vi "ATR.vi"() -> ()   [LabVIEW 2017]
panel:
  out "ATR 2":string[][](table)=[["Test Communication", "-", "-", "-", "-", ""], ["Set S/N", "-", "-", "-", "-", ""], ["Set Board Number", "-", "-", "-", "-", ""], [" ", "", "", "", "", ""], ["Test Communication", "-", "-", "-", "-", ""], ["Get S/N", "-", "-", "-", "", ""], ["Get Board Number", "-", "-", "-", "", ""], ["Get FW", "-", "-", "-", "", ""], ["Enable Motor", "", "", "", "", ""], ["Small position command", "", "", "", "", ""], ["Measure delta", "", "", "", "", ""], ["Velocity command", "", "", "", "", ""]] caption="ATR"
  out "ATR":string[][](table)=[["Test Communication", "-", "-", "-", "-", ""], ["Set S/N", "-", "-", "-", "-", ""], ["Set Board Number", "-", "-", "-", "-", ""], [" ", "", "", "", "", ""], ["Test Communication", "-", "-", "-", "-", ""], ["Get S/N", "-", "-", "-", "", ""], ["Get Board Number", "-", "-", "-", "", ""], ["Get FW", "-", "-", "-", "", ""], ["Enable Motor", "", "", "", "", ""], ["Small position command", "", "", "", "", ""], ["Measure delta", "", "", "", "", ""], ["Velocity command", "", "", "", "", ""]]
  out "Array 2":string[](array[string])
  out "Array":string[](array[string])
  out "deleted portion 2":string[](array[string])
  out "deleted portion":string[](array[string])
  out "ArrAHU":string[][](array[string])
  out "ArrEbay":string[][](array[string])
  out "Mort Temp":string[][](array[string])
  out "Aux":string[][](array[string])
  out "Burnin":string[][](array[string])
  out "Temp Algo":string[][](array[string])
  out "Speed":string[][](array[string])
  out "Tempreature calibration":string[][](array[string])
  out "StopTime":string[][](array[string])
  out "Enable":string[][](array[string])
  out "Communication":string[][](array[string])
  out "Visual Inspection":string[][](array[string])
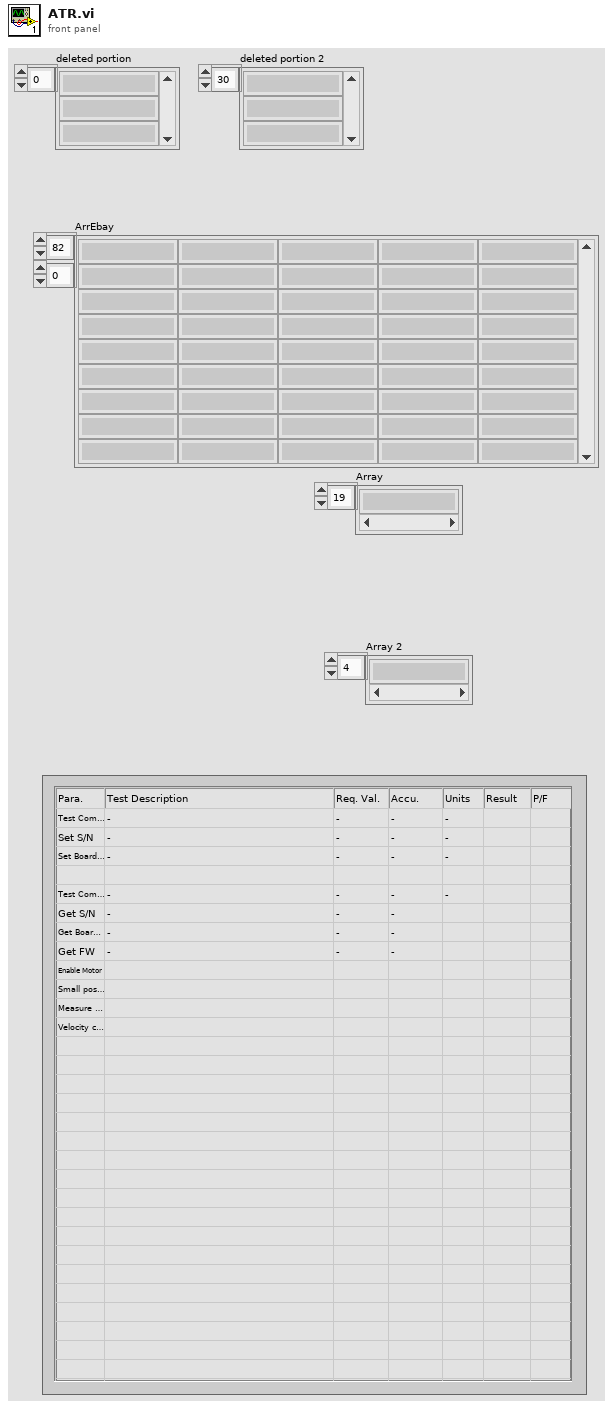
[diagram p1: front panel]
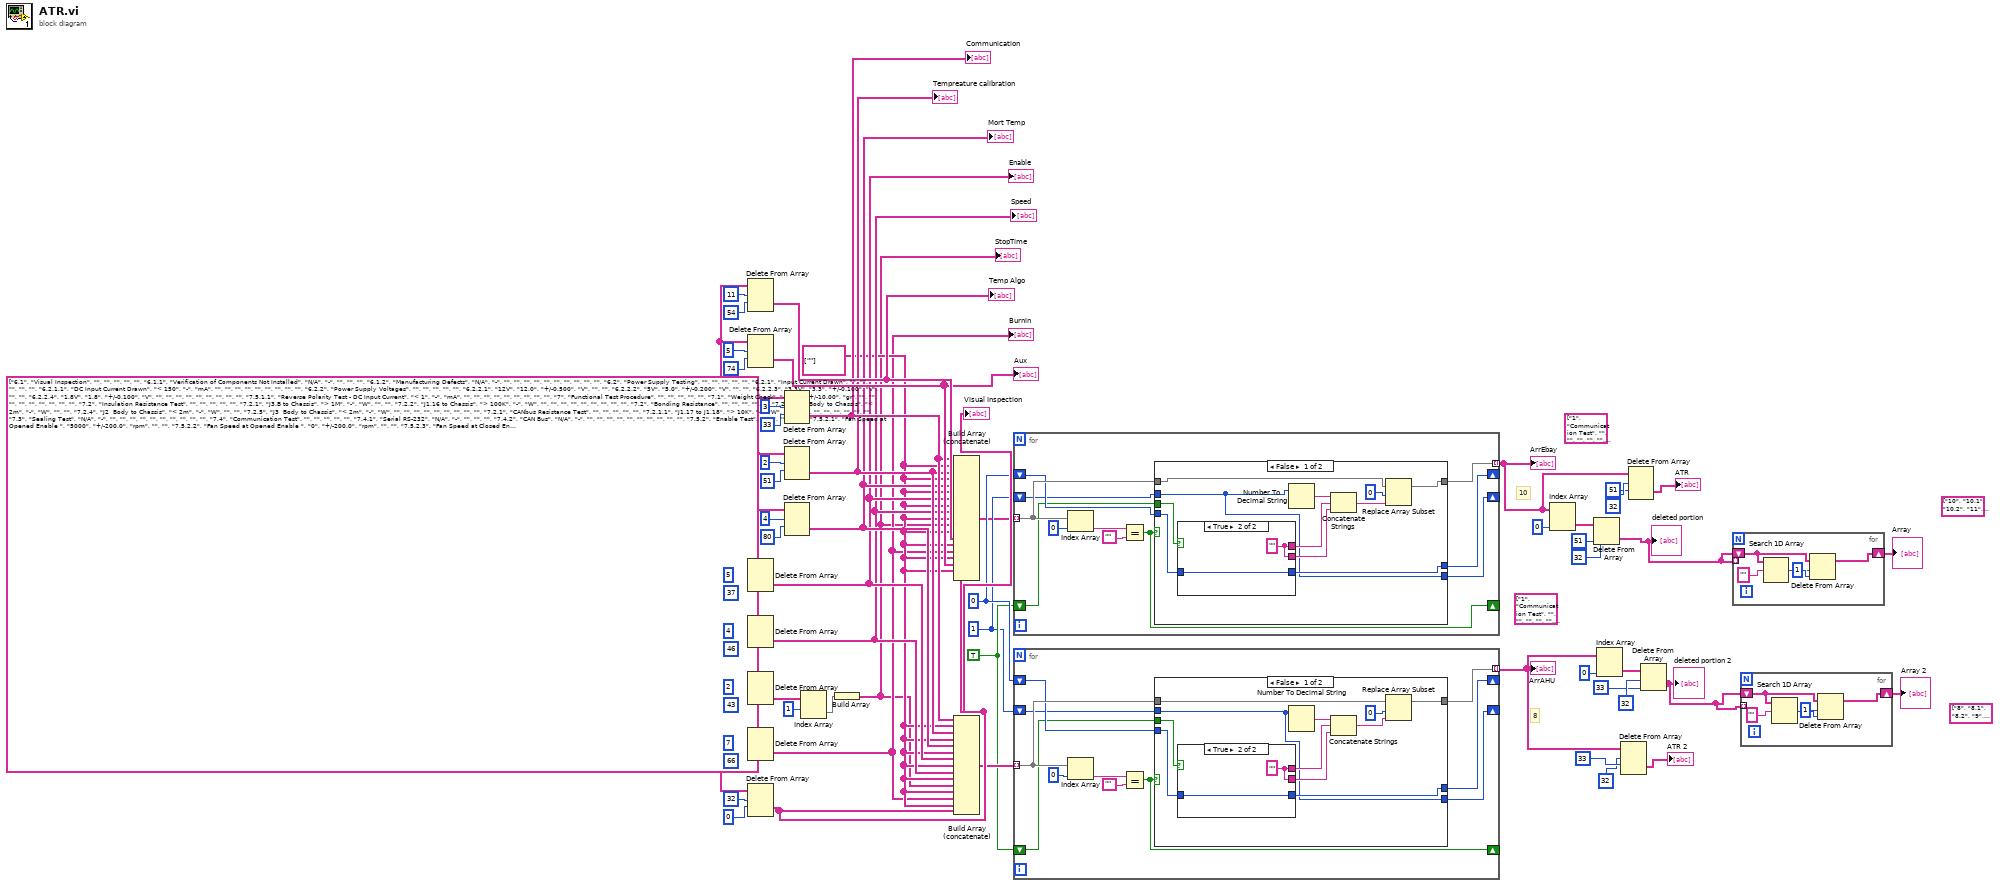
[diagram p0: block diagram]
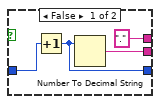
[diagram p2: hidden frame]
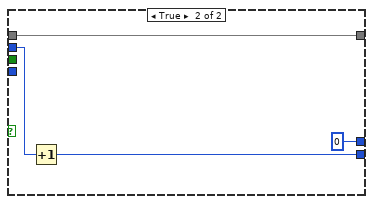
[diagram p3: hidden frame]
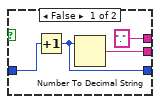
[diagram p4: hidden frame]
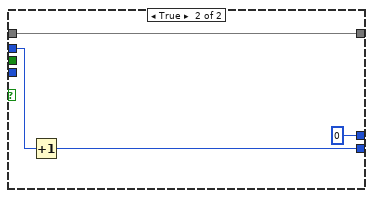
[diagram p5: hidden frame]
diagram:
  (unwired) string[] ["8", "8.1", "8.2", "9", "9.1", "9.2", "10", "10.1", "10.2", "10.3", "10.4", "11", "12", "12.1", "13", "13.1", "13.2", "14", "14.1", "14.2", "14.3", "15", "15.1", "16"] ("Array 3")
  (unwired) string[] ["10", "10.1", "10.2", "11", "11.1", "11.2", "12", "12.1", "12.2", "12.3", "12.4", "13", "14", "14.1", "15", "15.1", "15.2", "16", "16.1", "16.2", "16.3", "17", "17.1", "18"] ("Array 4")
  (unwired) string[][] [["1", "Communication Test", "", "", "", "", ""], ["1.1", "Serial RS-232", "N/A", "-", "", "", ""], ["1.2", "CAN Bus", "N/A", "-", "", "", ""], ["", "", "", "", "", "", ""], ["2", "Temperature Sensor Calibration", "", "", "", "", ""], ["2.1", "Sensor Reading Analog Offset", "0", "+/-0.100", ".", "", ""], ["", "", "", "", "", "", ""], ["3", "Motor Termistor Input Test", "", "", "", "", ""], ["3.1", "60 Degree", "60", "+/-3.00", "C", "", ""], ["3.2", "90 Degree", "90", "+/-3.00", "C", "", ""], ["3.3", "120 Degree", "120", "+/-3.00", "C", "", ""], ["", "", "", "", "", "", ""], ["4", "Enable Test", "", "", "", "", ""], ["4.1", "Fan Speed at Opened Enable ", "5000", "+/-200.0", "rpm", "", ""], ["4.2", "Fan Speed at Opened Enable ", "0", "+/-200.0", "rpm", "", ""], ["4.3", "Fan Speed at Closed Enable ", "5000", "+/-200.0", "rpm", "", ""], ["4.4", "Motor Rotation Direction", "Counter-clockwise (Inlet)", "-", "", "", ""], ["", "", "", "", "", "", ""], ["5", "Speed Command Test", "", "", "", "", ""], ["5.1", "Fan Speed", "6000", "+/-200.0", "rpm", "", ""], ["5.2", "Fan Speed", "11500", "+/-200.0", "rpm", "", ""], ["5.3", "Fan Speed", "15100", "+/-200.0", "rpm", "", ""], ["", "", "", "", "", "", ""], ["6", "Motor Stop time", "< 50", "-", "sec", "", ""], ["", "", "", "", "", "", ""], ["7", "Temperature Control Algorithm Test", "", "", "", "", ""], ["7.1", "Tair <   68 ± 2 oC", "6000", "+/-200.0", "rpm", "", ""], ["7.2", "Measured Temp.", "", "", "C", "", ""], ["7.3", "Tair >= 68 ± 2 oC", "11500", "+/-200.0", "rpm", "", ""], ["7.4", "Transition Temp.", "", "", "C", "", ""], ["7.5", "Tair >= 88 ± 2 oC", "15100", "+/-400.0", "rpm", "", ""], ["7.6", "Transition Temp.", "", "", "C", "", ""], ["7.7", "Tair <= 80 ± 2 oC", "11500", "+/-200.0", "rpm", "", ""], ["7.8", "Transition Temp.", "", "", "C", "", ""], ["7.9", "Tair <= 60 ± 2 oC", "6000", "+/-200.0", "rpm", "", ""], ["7.10", "Transition Temp.", "", "", "C", "", ""], ["", "", "", "", "", "", ""], ["8", "Burn-in Test", "", "", "", "", ""], ["8.1", "DC Input Current", "50", "+/-5.000", "A", "", ""], ["8.2", "Fan Speed", "15100", "+/-200.0", "rpm", "", ""], ["8.3", "Ambient Temperature", "25", "+/-13.00", "C", "", ""], ["8.4", "After 10 min of operation", "", "-", "C", "", ""], ["8.5", "After 20 min of operation", "", "-", "C", "", ""], ["8.6", "After 30 min of operation", "", "-", "C", "", ""], ["", "", "", "", "", "", ""], ["9", "Auxiliary Fan Test", "", "", "", "", ""], ["9.1", "Auxiliary Cooling Fan ON", "60", "+/-2.00", "C", "", ""], ["9.2", "Fan status", "ON", "-", "-", "", ""], ["9.3", "Auxiliary Cooling Fan OFF", "55", "+/-2.00", "C", "", ""], ["9.4", "Fan status", "OFF", "-", "-", "", ""], ["", "", "", "", "", "", ""], ["10", "Visual Inspection", "", "", "", "", ""], ["10.1", "Verification of Components Not Installed", "N/A", "-", "", "", ""], ["10.2", "Manufacturing Defects", "N/A", "-", "", "", ""], ["", "", "", "", "", "", ""], ["11", "Power Supply Testing", "", "", "", "", ""], ["11.1", "Input Current Drawn", "", "", "", "", ""], ["11.2", "DC Input Current", "< 150", "-", "mA", "", ""], ["", "", "", "", "", "", ""], ["12", "Power Supply Voltages", "", "", "", "", ""], ["12.1", "12V", "12.0", "+/-0.500", "V", "", ""], ["12.2", "5V", "5.0", "+/-0.200", "V", "", ""], ["12.3", "3.3V", "3.3", "+/-0.100", "V", "", ""], ["12.4", "1.8V", "1.8", "+/-0.100", "V", "", ""], ["", "", "", "", "", "", ""], ["13", "Reverse Polarity Test - DC Input Current", "< 1", "-", "mA", "", ""], ["", "", "", "", "", "", ""], ["14", "Functional Test Procedure", "", "", "", "", ""], ["14.1", "Weight Check", "4180", "+/-10.00", "gr", "", ""], ["", "", "", "", "", "", ""], ["15", "Insulation Resistance Test", "", "", "", "", ""], ["15.1", "J3.B to Chassis", "> 1M", "-", "W", "", ""], ["15.2", "J1.16 to Chassis", "> 100K", "-", "W", "", ""], ["", "", "", "", "", "", ""], ["16", "Bonding Resistance", "", "", "", "", ""], ["16.1", "J1 Body to Chassis", "< 2m", "-", "W", "", ""], ["16.2", "J2  Body to Chassis", "< 2m", "-", "W", "", ""], ["16.3", "J3  Body to Chassis", "< 2m", "-", "W", "", ""], ["", "", "", "", "", "", ""], ["17", "CANbus Resistance Test", "", "", "", "", ""], ["17.1", "J1.17 to J1.18", "> 10K", "-", "W", "", ""], ["", "", "", "", "", "", ""], ["18", "Sealing Test", "N/A", "-", "", "", ""]] ("ArrEbay 2")
  (unwired) string[][] [["1", "Communication Test", "", "", "", "", ""], ["1.1", "Serial RS-232", "N/A", "-", "", "", ""], ["1.2", "CAN Bus", "N/A", "-", "", "", ""], ["", "", "", "", "", "", ""], ["2", "Temperature Sensor Calibration", "", "", "", "", ""], ["2.1", "Sensor Reading Analog Offset", "0", "+/-0.100", ".", "", ""], ["", "", "", "", "", "", ""], ["3", "Motor Termistor Input Test", "", "", "", "", ""], ["3.1", "60 Degree", "60", "+/-3.00", "C", "", ""], ["3.2", "90 Degree", "90", "+/-3.00", "C", "", ""], ["3.3", "120 Degree", "120", "+/-3.00", "C", "", ""], ["", "", "", "", "", "", ""], ["4", "Enable Test", "", "", "", "", ""], ["4.1", "Fan Speed at Opened Enable ", "5000", "+/-200.0", "rpm", "", ""], ["4.2", "Fan Speed at Opened Enable ", "0", "+/-200.0", "rpm", "", ""], ["4.3", "Fan Speed at Closed Enable ", "5000", "+/-200.0", "rpm", "", ""], ["4.4", "Motor Rotation Direction", "Counter-clockwise (Inlet)", "-", "", "", ""], ["", "", "", "", "", "", ""], ["5", "Speed Command Test", "", "", "", "", ""], ["5.1", "Fan Speed", "6000", "+/-200.0", "rpm", "", ""], ["5.2", "Fan Speed", "11500", "+/-200.0", "rpm", "", ""], ["5.3", "Fan Speed", "15100", "+/-200.0", "rpm", "", ""], ["", "", "", "", "", "", ""], ["6", "Motor Stop time", "< 50", "-", "sec", "", ""], ["", "", "", "", "", "", ""], ["7", "Burn-in Test", "", "", "", "", ""], ["7.1", "DC Input Current", "50", "+/-5.000", "A", "", ""], ["7.2", "Fan Speed", "15100", "+/-200.0", "rpm", "", ""], ["7.3", "Ambient Temperature", "25", "+/-13.00", "C", "", ""], ["7.4", "After 10 min of operation", "", "-", "C", "", ""], ["7.5", "After 20 min of operation", "", "-", "C", "", ""], ["7.6", "After 30 min of operation", "", "-", "C", "", ""], ["", "", "", "", "", "", ""], ["8", "Visual Inspection", "", "", "", "", ""], ["8.1", "Verification of Components Not Installed", "N/A", "-", "", "", ""], ["8.2", "Manufacturing Defects", "N/A", "-", "", "", ""], ["", "", "", "", "", "", ""], ["9", "Power Supply Testing", "", "", "", "", ""], ["9.1", "Input Current Drawn", "", "", "", "", ""], ["9.2", "DC Input Current", "< 150", "-", "mA", "", ""], ["", "", "", "", "", "", ""], ["10", "Power Supply Voltages", "", "", "", "", ""], ["10.1", "12V", "12.0", "+/-0.500", "V", "", ""], ["10.2", "5V", "5.0", "+/-0.200", "V", "", ""], ["10.3", "3.3V", "3.3", "+/-0.100", "V", "", ""], ["10.4", "1.8V", "1.8", "+/-0.100", "V", "", ""], ["", "", "", "", "", "", ""], ["11", "Reverse Polarity Test - DC Input Current", "< 1", "-", "mA", "", ""], ["", "", "", "", "", "", ""], ["12", "Functional Test Procedure", "", "", "", "", ""], ["12.1", "Weight Check", "4180", "+/-10.00", "gr", "", ""], ["", "", "", "", "", "", ""], ["13", "Insulation Resistance Test", "", "", "", "", ""], ["13.1", "J3.B to Chassis", "> 1M", "-", "W", "", ""], ["13.2", "J1.16 to Chassis", "> 100K", "-", "W", "", ""], ["", "", "", "", "", "", ""], ["14", "Bonding Resistance", "", "", "", "", ""], ["14.1", "J1 Body to Chassis", "< 2m", "-", "W", "", ""], ["14.2", "J2  Body to Chassis", "< 2m", "-", "W", "", ""], ["14.3", "J3  Body to Chassis", "< 2m", "-", "W", "", ""], ["", "", "", "", "", "", ""], ["15", "CANbus Resistance Test", "", "", "", "", ""], ["15.1", "J1.17 to J1.18", "> 10K", "-", "W", "", ""], ["", "", "", "", "", "", ""], ["16", "Sealing Test", "N/A", "-", "", "", ""]] ("ArrAHU 2")
  w31 = string[][] [[""]] ("array")
  w28 = TRUE
  w27 = 1
  w29 = 0
  w39 = string[][] [["6.1", "Visual Inspection", "", "", "", "", ""], ["6.1.1", "Verification of Components Not Installed", "N/A", "-", "", "", ""], ["6.1.2", "Manufacturing Defects", "N/A", "-", "", "", ""], ["", "", "", "", "", "", ""], ["6.2", "Power Supply Testing", "", "", "", "", ""], ["6.2.1", "Input Current Drawn", "", "", "", "", ""], ["6.2.1.1", "DC Input Current Drawn", "< 150", "-", "mA", "", ""], ["", "", "", "", "", "", ""], ["6.2.2", "Power Supply Voltages", "", "", "", "", ""], ["6.2.2.1", "12V", "12.0", "+/-0.500", "V", "", ""], ["6.2.2.2", "5V", "5.0", "+/-0.200", "V", "", ""], ["6.2.2.3", "3.3V", "3.3", "+/-0.100", "V", "", ""], ["6.2.2.4", "1.8V", "1.8", "+/-0.100", "V", "", ""], ["", "", "", "", "", "", ""], ["7.5.1.1", "Reverse Polarity Test - DC Input Current", "< 1", "-", "mA", "", ""], ["", "", "", "", "", "", ""], ["7", "Functional Test Procedure", "", "", "", "", ""], ["7.1", "Weight Check", "4180", "+/-10.00", "gr", "", ""], ["", "", "", "", "", "", ""], ["7.2", "Insulation Resistance Test", "", "", "", "", ""], ["7.2.1", "J3.B to Chassis", "> 1M", "-", "W", "", ""], ["7.2.2", "J1.16 to Chassis", "> 100K", "-", "W", "", ""], ["", "", "", "", "", "", ""], ["7.2", "Bonding Resistance", "", "", "", "", ""], ["7.2.3", "J1 Body to Chassis", "< 2m", "-", "W", "", ""], ["7.2.4", "J2  Body to Chassis", "< 2m", "-", "W", "", ""], ["7.2.5", "J3  Body to Chassis", "< 2m", "-", "W", "", ""], ["", "", "", "", "", "", ""], ["7.2.1", "CANbus Resistance Test", "", "", "", "", ""], ["7.2.1.1", "J1.17 to J1.18", "> 10K", "-", "W", "", ""], ["", "", "", "", "", "", ""], ["7.3", "Sealing Test", "N/A", "-", "", "", ""], ["", "", "", "", "", "", ""], ["7.4", "Communication Test", "", "", "", "", ""], ["7.4.1", "Serial RS-232", "N/A", "-", "", "", ""], ["7.4.2", "CAN Bus", "N/A", "-", "", "", ""], ["", "", "", "", "", "", ""], ["7.5.2", "Enable Test", "", "", "", "", ""], ["7.5.2.1", "Fan Speed at Opened Enable ", "5000", "+/-200.0", "rpm", "", ""], ["7.5.2.2", "Fan Speed at Opened Enable ", "0", "+/-200.0", "rpm", "", ""], ["7.5.2.3", "Fan Speed at Closed Enable ", "5000", "+/-200.0", "rpm", "", ""], ["7.5.2.4", "Motor Rotation Direction", "Counter-clockwise (Inlet)", "-", "", "", ""], ["", "", "", "", "", "", ""], ["7.5.3", "Stop Time Test ", "", "", "", "", ""], ["7.5.3.1", "Motor Stop time", "< 50", "-", "sec", "", ""], ["", "", "", "", "", "", ""], ["7.5.4", "Speed Command Test", "", "", "", "", ""], ["7.5.4.1", "Fan Speed", "6000", "+/-200.0", "rpm", "", ""], ["7.5.4.2", "Fan Speed", "11500", "+/-200.0", "rpm", "", ""], ["7.5.4.3", "Fan Speed", "15100", "+/-200.0", "rpm", "", ""], ["", "", "", "", "", "", ""], ["7.5.5", "Temperature Sensor Calibration", "", "", "", "", ""], ["7.5.5.1", "Sensor Reading Analog Offset", "0", "+/-0.100", ".", "", ""], ["", "", "", "", "", "", ""], ["7.5.6", "Temperature Control Algorithm Test", "", "", "", "", ""], ["7.5.6.1", "Tair <   68 ± 2 oC", "6000", "+/-200.0", "rpm", "", ""], ["7.5.6.2", "Measured Temp.", "", "", "C", "", ""], ["7.5.6.3", "Tair >= 68 ± 2 oC", "11500", "+/-200.0", "rpm", "", ""], ["7.5.6.4", "Transition Temp.", "", "", "C", "", ""], ["7.5.6.5", "Tair >= 88 ± 2 oC", "15100", "+/-400.0", "rpm", "", ""], ["7.5.6.6", "Transition Temp.", "", "", "C", "", ""], ["7.5.6.7", "Tair <= 80 ± 2 oC", "11500", "+/-200.0", "rpm", "", ""], ["7.5.6.8", "Transition Temp.", "", "", "C", "", ""], ["7.5.6.9", "Tair <= 60 ± 2 oC", "6000", "+/-200.0", "rpm", "", ""], ["7.5.6.10", "Transition Temp.", "", "", "C", "", ""], ["", "", "", "", "", "", ""], ["7.5.7", "Burn-in Test", "", "", "", "", ""], ["7.5.7.1", "DC Input Current", "50", "+/-5.000", "A", "", ""], ["7.5.7.2", "Fan Speed", "15100", "+/-200.0", "rpm", "", ""], ["7.5.7.3", "Ambient Temperature", "25", "+/-13.00", "C", "", ""], ["7.5.7.4", "After 10 min of operation", "", "-", "C", "", ""], ["7.5.7.5", "After 20 min of operation", "", "-", "C", "", ""], ["7.5.7.6", "After 30 min of operation", "", "-", "C", "", ""], ["", "", "", "", "", "", ""], ["8", "Auxiliary Fan Test", "", "", "", "", ""], ["8.1", "Auxiliary Cooling Fan ON", "60", "+/-2.00", "C", "", ""], ["8.2", "Fan status", "ON", "-", "-", "", ""], ["8.3", "Auxiliary Cooling Fan OFF", "55", "+/-2.00", "C", "", ""], ["8.4", "Fan status", "OFF", "-", "-", "", ""], ["", "", "", "", "", "", ""], ["9", "Motor Termistor Input Test", "", "", "", "", ""], ["9.1", "60 Degree", "60", "+/-3.00", "C", "", ""], ["9.2", "90 Degree", "90", "+/-3.00", "C", "", ""], ["9.3", "120 Degree", "120", "+/-3.00", "C", "", ""]] ("data")
  # "8"
  # "10"
  n1 = Delete From Array(array=w39, length=11, index (row)=54) -> (deleted portion=w38:string[][])  [unwired: 1 in, 1 out]
  "Temp Algo" <- w38
  n2 = Delete From Array(array=w39, length=5, index (row)=74) -> (deleted portion=w37:string[][])  [unwired: 1 in, 1 out]
  "Aux" <- w37
  n3 = Delete From Array(array=w39, length=5, index (row)=37) -> (deleted portion=w33:string[][])  [unwired: 1 in, 1 out]
  "Enable" <- w33
  n4 = Delete From Array(array=w39, length=4, index (row)=46) -> (deleted portion=w32:string[][])  [unwired: 1 in, 1 out]
  "Speed" <- w32
  n5 = Delete From Array(array=w39, length=2, index (row)=43) -> (deleted portion=w24:string[][])  [unwired: 1 in, 1 out]
  n6 = Delete From Array(array=w39, length=7, index (row)=66) -> (deleted portion=w25:string[][])  [unwired: 1 in, 1 out]
  "Burnin" <- w25
  n7 = Delete From Array(array=w39, length=32, index (row)=0) -> (deleted portion=w46:string[][])  [unwired: 1 in, 1 out]
  "Visual Inspection" <- w46
  n8 = Delete From Array(array=w39, length=3, index (row)=33) -> (deleted portion=w36:string[][])  [unwired: 1 in, 1 out]
  "Communication" <- w36
  n9 = Delete From Array(array=w39, length=2, index (row)=51) -> (deleted portion=w35:string[][])  [unwired: 1 in, 1 out]
  "Tempreature calibration" <- w35
  n10 = Delete From Array(array=w39, length=4, index (row)=80) -> (deleted portion=w34:string[][])  [unwired: 1 in, 1 out]
  "Mort Temp" <- w34
  n11 = Index Array(array=w24, index (row)=1) -> (element=w22:string[])  [unwired: 1 in]
  n12 = Build Array(w22) -> (w21:string[][])
  "StopTime" <- w21
  n13 = Build Array (concatenate)(w36, w31, w35, w31, w34, w31, w33, w31, w32, w31, w21, w31, w38, w31, w25, w31, w37, w31, w46) -> (w26:string[][])
  n14 = Build Array (concatenate)(w36, w31, w35, w31, w34, w31, w33, w31, w32, w31, w21, w31, w25, w31, w46) -> (w30:string[][])
  n15 = for {
    tunnel: w26 -> [w70] mode=indexing
    tunnel: [w71] -> w6 mode=indexing
    shift-right: [w65] -> _
    shift-left: w29 -> [w66]
    shift-right: [w63] -> _
    shift-left: w27 -> [w64]
    shift-right: [w62] -> _
    shift-left: w28 -> [w61]
    n16 = Index Array(array=w70, index=0) -> (element=w68:string)
    n17 = Equal?(x=w68, y="") -> (x = y?=w62:bool)
    n18 = case shown="False" w62 {
      tunnel: w66 -> [w76 _]
      tunnel: [w79 w92] -> w71
      tunnel: w70 -> [w78 w92]
      tunnel: [w77 0] -> w65
      tunnel: w64 -> [w73 w91]
      tunnel: [w73 w90] -> w63
      tunnel: w61 -> [w72 _]
      frame False {
        n19 = case shown="True" w72 {
          tunnel: [w86 w88] -> w81
          tunnel: [w85 w87] -> w77
          tunnel: w76 -> [w84 w87]
          tunnel: ["." ("string") w88] -> w74
          frame False {
            n20 = Increment(x=w84) -> (x+1=w85:i32)
            n21 = Number To Decimal String(number=w85) -> (decimal integer string=w86:string)  [unwired: 1 in]
          }
          frame True {
            w88 = "" ("string")
          }
        }
        n22 = Number To Decimal String(number=w73) -> (decimal integer string=w75:string)  [unwired: 1 in]
        n23 = Concatenate Strings(w75, w74, w81) -> (w80:string)
        n24 = Replace Array Subset(array=w78, new element=w80, index=0) -> (w79:string[])
      }
      frame True {
        n25 = Increment(x=w91) -> (x+1=w90:i32)
      }
    }
  }
  "ArrEbay" <- w6
  n26 = for {
    tunnel: w30 -> [w102] mode=indexing
    tunnel: [w103] -> w1 mode=indexing
    shift-right: [w97] -> _
    shift-left: w29 -> [w98]
    shift-right: [w95] -> _
    shift-left: w27 -> [w96]
    shift-right: [w94] -> _
    shift-left: w28 -> [w93]
    n27 = Index Array(array=w102, index=0) -> (element=w100:string)
    n28 = Equal?(x=w100, y="") -> (x = y?=w94:bool)
    n29 = case shown="False" w94 {
      tunnel: w98 -> [w108 _]
      tunnel: [w111 w124] -> w103
      tunnel: w102 -> [w110 w124]
      tunnel: [w109 0] -> w97
      tunnel: w96 -> [w105 w123]
      tunnel: [w105 w122] -> w95
      tunnel: w93 -> [w104 _]
      frame False {
        n30 = case shown="True" w104 {
          tunnel: [w118 w120] -> w113
          tunnel: [w117 w119] -> w109
          tunnel: w108 -> [w116 w119]
          tunnel: ["." ("string") w120] -> w106
          frame False {
            n31 = Increment(x=w116) -> (x+1=w117:i32)
            n32 = Number To Decimal String(number=w117) -> (decimal integer string=w118:string)  [unwired: 1 in]
          }
          frame True {
            w120 = "" ("string")
          }
        }
        n33 = Number To Decimal String(number=w105) -> (decimal integer string=w107:string)  [unwired: 1 in]
        n34 = Concatenate Strings(w107, w106, w113) -> (w112:string)
        n35 = Replace Array Subset(array=w110, new element=w112, index=0) -> (w111:string[])
      }
      frame True {
        n36 = Increment(x=w123) -> (x+1=w122:i32)
      }
    }
  }
  "ArrAHU" <- w1
  n37 = Index Array(array=w6, index (col)=0 ("disabled index (col)")) -> (element=w19:string[])  [unwired: 1 in]
  n38 = Delete From Array(array=w19, length=32, index=51) -> (deleted portion=w12:string[])  [unwired: 1 out]
  "deleted portion" <- w12
  n39 = Index Array(array=w1, index (col)=0 ("disabled index (col)")) -> (element=w14:string[])  [unwired: 1 in]
  n40 = Delete From Array(array=w1, length=32, index (row)=33 ("index")) -> (deleted portion=→"ATR 2":string[][])  [unwired: 1 in, 1 out]
  n41 = Delete From Array(array=w6, length=32, index (row)=51 ("index")) -> (deleted portion=→"ATR":string[][])  [unwired: 1 in, 1 out]
  n42 = Delete From Array(array=w14, length=32, index=33) -> (deleted portion=w9:string[])  [unwired: 1 out]
  "deleted portion 2" <- w9
  n43 = for {
    tunnel: w12 -> [_] mode=indexing
    shift-right: [w125] -> w11
    shift-left: w12 -> [w128]
    n44 = Search 1D Array(1D array=w128, element="") -> (index of element=w127:i32)  [unwired: 1 in]
    n45 = Delete From Array(array=w128, length=1, index=w127) -> (array with subset deleted=w125:string[])  [unwired: 1 out]
  }
  "Array" <- w11
  n46 = for {
    shift-right: [w130] -> w10
    shift-left: w9 -> [w133]
    tunnel: w9 -> [_] mode=indexing
    n47 = Search 1D Array(1D array=w133, element="") -> (index of element=w132:i32)  [unwired: 1 in]
    n48 = Delete From Array(array=w133, length=1, index=w132) -> (array with subset deleted=w130:string[])  [unwired: 1 out]
  }
  "Array 2" <- w10
